vi "To ID (SubVI).vi"(10 "element":T1) -> (2 "ID":T2)   [LabVIEW 2021]
uses:
  controls/ID.ctl
  controls/ID Selector.ctl
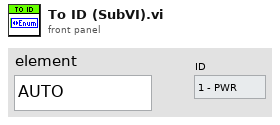
[diagram p1: front panel]
types:
  T1 = typedef "ID Selector.ctl" = enum16{"AUTO", "1 - PWR", "2 - SM", "3 - DC", "4 - DM", "5 - WS", "6 - DS", "7 - WC", "8 - WA", "9 - WM", "10 - DA", "11 - WH", "12 - DH"}
  T2 = typedef "ID.ctl" = enum16{"1 - PWR", "2 - SM", "3 - DC", "4 - DM", "5 - WS", "6 - DS", "7 - WC", "8 - WA", "9 - WM", "10 - DA", "11 - WH", "12 - DH"}
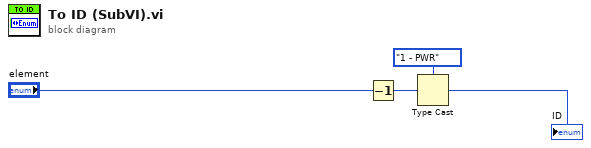
[diagram p0: block diagram]
diagram:
  n1 = Decrement(x="element") -> (x-1=w4:T1)
  n2 = Type Cast(type=ID."1 - PWR" ("ID"), x=w4) -> (*(type *) &x=→"ID":T2)
